vi "rethinkdb_hashlib_scram_client_final.vi"(9 "password":string, 10 "server_first_message":string, 11 "client_first_message":string) -> (3 "client_final_message":string)   [LabVIEW 2017]
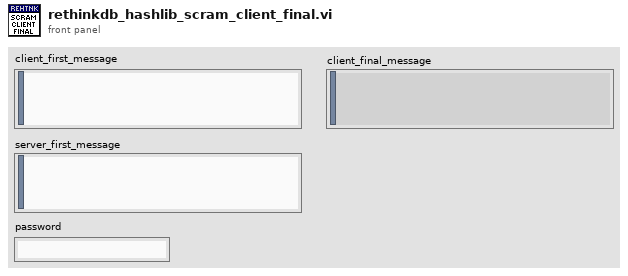
[diagram p1: front panel]
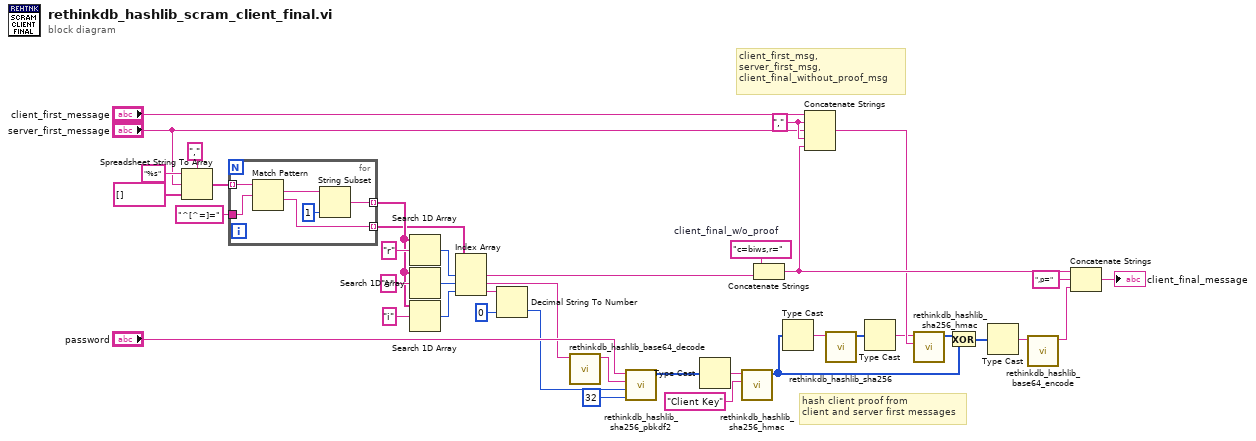
[diagram p0: block diagram]
diagram:
  w33 = "," ("string")
  w32 = "c=biws,r="  # client_final_w/o_proof
  # "hash client proof from \nclient and server first messages"
  # "client_first_msg,\nserver_first_msg,\nclient_final_without_proof_msg"
  n1 = Spreadsheet String To Array(delimiter (Tab)=",", format string="%s", spreadsheet string="server_first_message", array type (2D Dbl)=string[] []) -> (array=w16:string[])
  n2 = for {
    tunnel: w16 -> [w46] mode=indexing
    tunnel: [w42] -> w2 mode=indexing
    tunnel: [w45] -> w1 mode=indexing
    tunnel: "^[^=]=" ("regular expression") -> [w44]
    n3 = Match Pattern(string=w46, regular expression=w44) -> (match substring=w41:string, after substring=w45:string)  [unwired: 1 in, 2 out]
    n4 = String Subset(string=w41, length (rest)=1 ("length (rest)")) -> (substring=w42:string)  [unwired: 1 in]
  }
  n5 = Search 1D Array(1D array=w2, element="r") -> (index of element=w12:i32)  [unwired: 1 in]
  n6 = Search 1D Array(1D array=w2, element="s") -> (index of element=w11:i32)  [unwired: 1 in]
  n7 = Search 1D Array(1D array=w2, element="i") -> (index of element=w9:i32)  [unwired: 1 in]
  n8 = Index Array(array=w1, index #1=w12, index #2=w11, index #3=w9) -> (element #1=w5:string, element #2=w4:string, element #3=w8:string)
  n9 = Decimal String To Number(string=w8, default (0L)=0 ("default (0 I32)")) -> (number=w3:i32)  [unwired: 1 in, 1 out]
  n10 = call "rethinkdb_hashlib_base64_decode.vi"("base64"=w4) -> ("string"=w20:string)  [unwired: 10 in]
  n11 = call "rethinkdb_hashlib_sha256_pbkdf2.vi"("dkLen (32octets=sha256)"=32 ("32octets=sha256"), "iterations"=w3, "salt"=w20, "password"="password") -> ("sha-256"=w28:u32[])  [unwired: 7 in]
  n12 = Type Cast(x=w28) -> (*(type *) &x=w30:string)  [unwired: 1 in]
  n13 = call "rethinkdb_hashlib_sha256_hmac.vi"("data"="Client Key" ("key"), "key"=w30) -> ("sha256"=w24:u32[])  [unwired: 9 in]
  n14 = Concatenate Strings(w32, w5) -> (w37:string)
  n15 = Type Cast(x=w24) -> (*(type *) &x=w21:string)  [unwired: 1 in]
  n16 = Concatenate Strings("client_first_message", w33, "server_first_message", w33, w37) -> (w34:string)
  n17 = call "rethinkdb_hashlib_sha256.vi"("data"=w21) -> ("sha256"=w22:u32[])  [unwired: 10 in]
  n18 = Type Cast(x=w22) -> (*(type *) &x=w29:string)  [unwired: 1 in]
  n19 = call "rethinkdb_hashlib_sha256_hmac.vi"("data"=w34, "key"=w29) -> ("sha256"=w23:u32[])  [unwired: 9 in]
  n20 = Exclusive Or(1:w24, 2:w23) -> (0:w25:u32[])
  n21 = Type Cast(x=w25) -> (*(type *) &x=w26:string)  [unwired: 1 in]
  n22 = call "rethinkdb_hashlib_base64_encode.vi"("string"=w26) -> ("base64"=w39:string)  [unwired: 10 in]
  n23 = Concatenate Strings(w37, ",p=", w39) -> (→"client_final_message":string)
